vi "Multirecord Acquisition (FPGA).vi"() -> ()   [LabVIEW 2021]
doc: "Use this VI as a template for the reconfigurable oscilloscope acquisition design. The block diagram is divided into three main loops.\n\nRegister Bus: This loop initializes the registers that are needed to support the configuration of the device. The FIFO bus, on the left, allows all the other design libraries to communicate with one another. This loop is very important to support the proper behavior of the instrument design library components.\n\nAcquisition: Acquires data from the I/O channels and writes the data into the record memory using the <B>Write</B> VI of the Multirecord Acquisition instrument design library. This VI also evaluates the various acquisition triggers and decides whether to acquire each data value in record memory. The host level VI (Fetch Record.vi) can read acquired records from the DRAM. The data is stored in 2 DRAM banks, each with 768 MB of storage.\n\nFetch: The recorded data is retrieved when the <B>Fetch Single Record</B> VI is run from the host VI. The <B>Write to Fetch DMA FIFO</B> VI writes data to the acq.fetch fifo 0 to transmit record data form the FPGA to the record fetch VIs on the host. This DMA FIFO must have a predefined name based on the instance parameter. By default, it is 0 (since the associated terminal on the <B>Create Resources DRAM Write Read</B> VI is unwired), so the connected FIFO is named acq.fetch fifo 0."
uses:
  Trigger/SubVIs/Types/Trigger Type.ctl
  <instrlib>/_niInstr/Data Trigger/v1/Shared/Public/Level Configuration FXP(+-,18,1).ctl
  <instrlib>/_niInstr/Data Trigger/v1/Shared/Public/Level Configuration Trigger When.ctl
  <instrlib>/_niInstr/Data Trigger/v1/Shared/Public/Edge Configuration FXP(+-,18,1).ctl
  <instrlib>/_niInstr/Data Trigger/v1/Shared/Public/Edge Configuration Trigger Slope.ctl
  FPGA Interface Typedefinitions/Trigger Combination Type.ctl
  <vilib>/Platform/TimedLoop/XDataNode/timing_clust.ctl
  <vilib>/Platform/TimedLoop/XDataNode/nitl_modes.ctl
  <vilib>/Platform/TimedLoop/XDataNode/wakeup.ctl
  <instrlib>/_niInstr/FIFO Register Bus/v1/FPGA/niInstr FIFO Register Bus v1 FPGA.lvclass
  C:/Program Files (x86)/National Instruments/LabVIEW 2021/instr.lib/_niInstr/Instruction Framework/v1/FPGA/Interfaces/Instruction Producer/Instruction Producer.lvclass
  <instrlib>/_niInstr/Multirecord Acquisition/Common/v1/FPGA/niInstr Multirecord Acquisition Common v1 FPGA.lvclass
  C:/Program Files (x86)/National Instruments/LabVIEW 2021/instr.lib/_niInstr/Multirecord Acquisition/Interface/v1/FPGA/niInstr Multirecord Acquisition v1 FPGA.lvclass
  <vilib>/rvi/Emulation/niFpgaSctlEmulationGetInTimedLoop.vi
  <vilib>/rvi/Emulation/niFpgaEmulationReportErrorSimple.vi
  <vilib>/rvi/Emulation/niFpgaGetClockAttributes.vi
  <vilib>/rvi/Emulation/niFpgaCriticalErrorInLSC.vi
  <instrlib>/_niInstr/Multirecord Acquisition/Common/v1/FPGA/Private/Create Fetch DMA FIFO Resources U8x32.vi
  <instrlib>/_niInstr/Multirecord Acquisition/Common/v1/FPGA/Private/Create Resources DRAM U384x2 U768 Write Read.vi
  <instrlib>/_niInstr/Multirecord Acquisition/Interface/v1/FPGA/Private/Retrieve Record U16 Wrapper.vi
  <instrlib>/_niInstr/Multirecord Acquisition/Interface/v1/FPGA/Private/Write to Fetch DMA FIFO U16 Wrapper.vi
  <vilib>/rvi/eio/common/nirviEmuTemplateMethod_errors.vi
  <instrlib>/HSAI-RIO/Config/Group A/v1/FPGA/Digital Correction/Validate 8 Channel Data.vi
  <instrlib>/HSAI-RIO/Config/Group A/v1/FPGA/Digital Correction/Digital Correction (8 Ch).vi
  <instrlib>/HSAI-RIO/Config/Group A/v1/FPGA/Digital Correction/FIR Filter (8 Ch).vi
  DSP/SubVIs/Integer decimationx8ch.vi
  Data Type Conversion/SubVIs/Remove Overflow FXP(+-,18,1)x8ch.vi
  <instrlib>/_niInstr/Channel/v1/FPGA/Private/Select/Select FXP(+-,18,1,)xNspcx8ch.vi
  Trigger/Trigger FXP(+,-,18,1).vi
  Data Type Conversion/SubVIs/Data Type Conversion FXP(+-,18,1) to I16x8ch.vi
  <instrlib>/_niInstr/Channel/v1/FPGA/Private/Select and Interleave/Select And Interleave I16xNspcx8ch.vi
  <instrlib>/_niInstr/Multirecord Acquisition/Interface/v1/FPGA/Private/Write I16 Wrapper.vi
  <vilib>/Platform/TimedLoop/XDataNode/XDataNode.xnode
  <vilib>/eio/EIONode/EIONode.xnode
  <instrlib>/_niInstr/Instruction Framework/v1/FPGA/Top Level Bus/Register Configuration/Register Configuration.lvclass
  <vilib>/Platform/TimedLoop/XDataNode/XDNodeRunTimeDep.lvlib
  <instrlib>/_niInstr/Multirecord Acquisition/Interface/v1/FPGA/niInstr Multirecord Acquisition v1 FPGA.lvclass
  <vilib>/rvi/LocalResourceManager/LocalResourceManager.xnode
  <vilib>/rvi/eio/common/nirviEmuReportErrorAndStop.vi
  <vilib>/rvi/DataTransferAndStorage/Container/Common/niFpgaContainerGetUniqueNameForEmu.vi
  <vilib>/rvi/DataTransferAndStorage/Container/Common/niFpgaContainerSetEmuInfo.vi
  <instrlib>/_niInstr/Channel/v1/FPGA/niInstr Channel v1 FPGA.lvlib
  <instrlib>/_niInstr/Basic Elements/v1/FPGA/niInstr Basic Elements v1 FPGA.lvlib
  <instrlib>/HSAI-RIO/Config/Group A/v1/FPGA/Digital Correction/Digital Correction.lvclass
  <instrlib>/HSAI-RIO/Config/Group A/v1/FPGA/Config Registers/Config Registers.lvclass
  <instrlib>/_niInstr/Data Trigger/v1/Shared/niInstr Data Trigger v1 Shared.lvlib
  Emulation/SubVIs/2 Element Generate Sine Cos Data FXP(+,-,14,1).vi
  C:/Program Files (x86)/National Instruments/LabVIEW 2021/instr.lib/_niInstr/Multirecord Acquisition/Common/v1/FPGA/niInstr Multirecord Acquisition Common v1 FPGA.lvclass
  <instrlib>/_niInstr/Multirecord Acquisition/Common/v1/FPGA/Private/Create Resources BRAM U384.vi
  <instrlib>/_niInstr/Multirecord Acquisition/Common/v1/FPGA/Private/Create Resources DRAM U384.vi
  <instrlib>/_niInstr/Multirecord Acquisition/Common/v1/FPGA/Private/Create Resources BRAM U768.vi
  FPGA Interface Typedefinitions/FPGA Interface Typedefinitions.lvlib
panel:
  in  "trigger.channel A":u8
  in  "trigger.rearm delay":u16=2
  in  "start trigger":bool=TRUE
  in  "reset":bool
  in  "trigger.combination type":T1
  in  "trigger.level B":T2
  in  "trigger.edge A":T4
  in  "trigger.level A":T2
  in  "trigger.type A":T6
  out "fifo reg bus data 0":u64
  out "fifo reg bus status 0":u32
  in  "fifo reg bus ctrl 0":u32
  out "overflow":bool
  in  "dsp.decimation factor":u16
  out "overload":bool
  in  "channel.enable mask":u16=65535 format="%.0b"
  in  "channel.number of channels":u8=8
  # "Register Bus Controls"
  # "FPGA"
  # "Acquisition Loop Controls"
  # "DSP"
  # "Trigger"
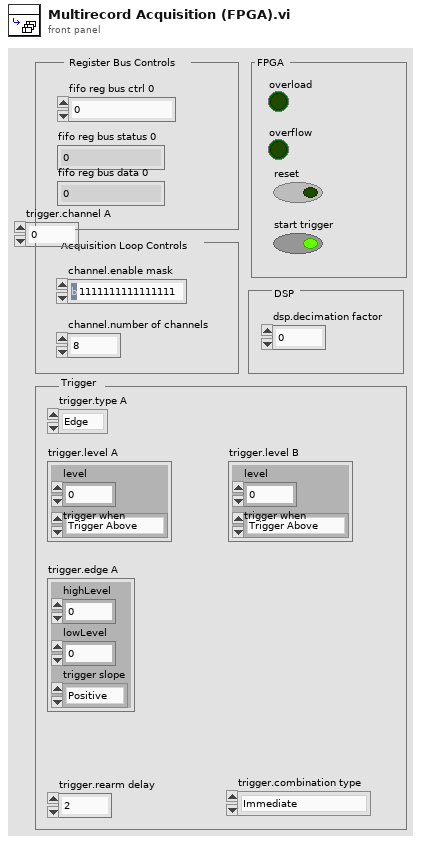
[diagram p1: front panel]
types:
  T1 = typedef "FPGA Interface Typedefinitions.lvlib/Trigger Combination Type.ctl" = enum16{"Immediate", "A", "B", "OR", "AND", "A THEN B", "B THEN A", "High Resolution"}
  T2 = typedef "niInstr Data Trigger v1 Shared.lvlib/Level Configuration FXP(+-,18,1).ctl" = cluster{"level":fxp<+/-,18,1>, "trigger when":T3}
  T3 = typedef "niInstr Data Trigger v1 Shared.lvlib/Level Configuration Trigger When.ctl" = enum8{"Trigger Above", "Trigger Below"}
  T4 = typedef "niInstr Data Trigger v1 Shared.lvlib/Edge Configuration FXP(+-,18,1).ctl" = cluster{"highLevel":fxp<+/-,18,1>, "lowLevel":fxp<+/-,18,1>, "trigger slope":T5}
  T5 = typedef "niInstr Data Trigger v1 Shared.lvlib/Edge Configuration Trigger Slope.ctl" = enum8{"Positive", "Negative"}
  T6 = typedef "Trigger Type.ctl" = enum16{"Edge", "Level", "Custom"}
  T7 = cluster{"memory 1":refnum<k21>, "memory 2":refnum<k21>}
  T8 = typedef "XDNodeRunTimeDep.lvlib/timing_clust.ctl" = cluster{"Expected End [f-1]":u64, "Actual End [f-1]":u64, "Finished Late? [f-1]":bool, "Expected End [i-1]":u64, "Actual End [i-1]":u64, "Finished Late? [i-1]":bool, "Expected Start [i]":u64, "Actual Start [i]":u64, "Expected Start [f]":u64, "Actual Start [f]":u64, "Source Name":string, "Structure Name":string, "Period":i64, "Deadline":i64, "Offset":i64, "Start":i64, "Priority":i32, "Timeout":i32, "Mode":T9, "Wakeup Reason":T10, "Error":errorcluster, "Source Type":string, "Secondary Source Type":string, "Global End Time":u64, "Global Start Time":u64, "Frame Duration":u64, "Iteration Duration":u64, "Assigned CPU":i32, "I/O Scan Engine Mode":u32}
  T9 = typedef "XDNodeRunTimeDep.lvlib/nitl_modes.ctl" = enum32{"No Change", "Process missed periods, maintain original phase", "Discard missed periods, maintain original phase", "Process missed periods, ignore original phase", "Discard missed periods, ignore original phase"}
  T10 = typedef "XDNodeRunTimeDep.lvlib/wakeup.ctl" = enum32{"Normal", "Aborted", "Asynchronous wakeup", "Timing source error", "Timed loop error", "Timeout"}
  T11 = cluster{"Channel 0":fxp<+/-,14,1>[], "Channel 1":fxp<+/-,14,1>[], "Channel 2":fxp<+/-,14,1>[], "Channel 3":fxp<+/-,14,1>[], "Channel 4":fxp<+/-,14,1>[], "Channel 5":fxp<+/-,14,1>[], "Channel 6":fxp<+/-,14,1>[], "Channel 7":fxp<+/-,14,1>[]}
  T12 = cluster{"Channel 0":fxp<+/-,18,1>[], "Channel 1":fxp<+/-,18,1>[], "Channel 2":fxp<+/-,18,1>[], "Channel 3":fxp<+/-,18,1>[], "Channel 4":fxp<+/-,18,1>[], "Channel 5":fxp<+/-,18,1>[], "Channel 6":fxp<+/-,18,1>[], "Channel 7":fxp<+/-,18,1>[]}
  T13 = cluster{"channel 0":fxp<+/-,18,1>[], "channel 1":fxp<+/-,18,1>[], "channel 2":fxp<+/-,18,1>[], "channel 3":fxp<+/-,18,1>[], "channel 4":fxp<+/-,18,1>[], "channel 5":fxp<+/-,18,1>[], "channel 6":fxp<+/-,18,1>[], "channel 7":fxp<+/-,18,1>[]}
  T14 = cluster{"channel 0":i16[], "channel 1":i16[], "channel 2":i16[], "channel 3":i16[], "channel 4":i16[], "channel 5":i16[], "channel 6":i16[], "channel 7":i16[]}
  T15 = typedef "niInstr Multirecord Acquisition v1 FPGA.lvclass/Timestamp.ctl" = cluster{"timestamp":u64, "valid":bool}
  T16 = typedef "niInstr Types v1 Shared.lvlib/Input Triggers.ctl" = cluster{"start":bool, "advance":bool, "reference":bool, "start trigger index":u16, "advance trigger index":u16, "reference trigger index":u16, "reference trigger correction cycle count":u32}
  T17 = typedef "niInstr Types v1 Shared.lvlib/Sample Format.ctl" = cluster{"bits per channel":u16, "samples per clock":u16, "channels":u8}
  T18 = typedef "niInstr Multirecord Acquisition v1 FPGA.lvclass/Events.ctl" = cluster{"ready for start":bool, "ready for advance":bool, "ready for reference":bool, "end of record":bool, "done":bool, "start trigger":bool, "advance trigger":bool, "reference trigger":bool, "start trigger index":u16, "advance trigger index":u16, "reference trigger index":u16}
  T19 = typedef "niInstr Multirecord Acquisition v1 FPGA.lvclass/Retrieve Data Info.ctl" = cluster{"read request size (bits)":u64, "valid data offset (bits)":u16, "valid data size (bits)":u16, "first sample of request":bool, "last sample of request":bool, "Token":T20}
  T20 = typedef "niInstr Types v1 Shared.lvlib/Token.ctl" = cluster{"identifier":u8, "value":u32}
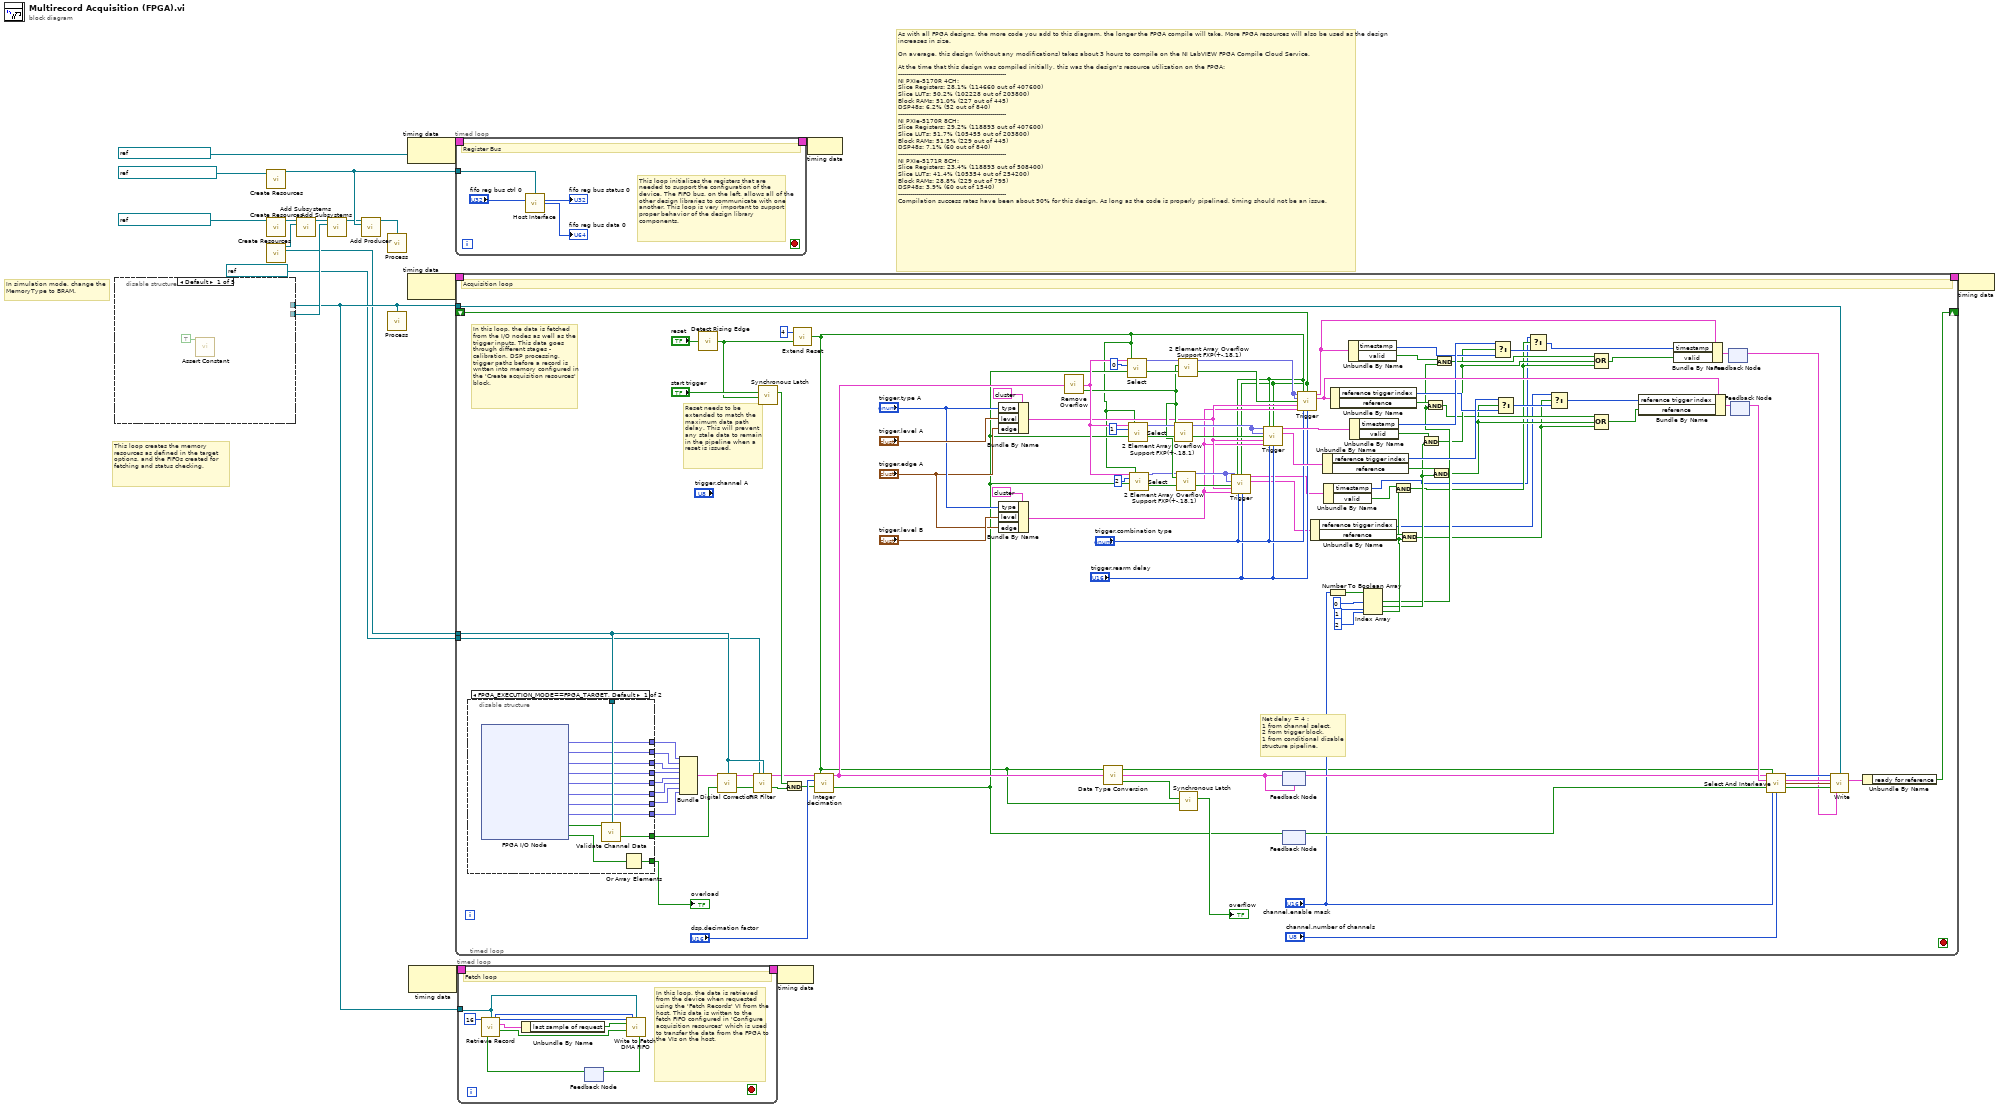
[diagram p0: block diagram]
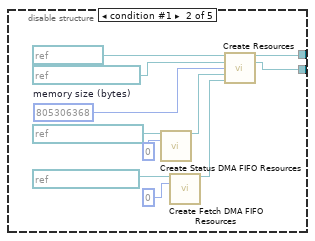
[diagram p2: hidden frame]
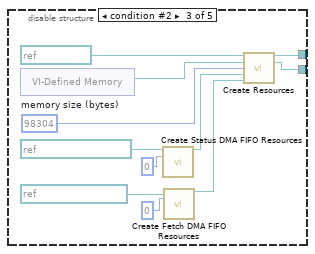
[diagram p3: hidden frame]
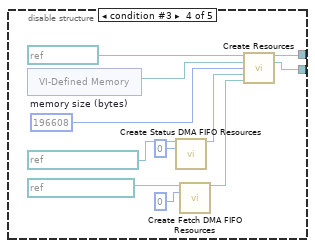
[diagram p4: hidden frame]
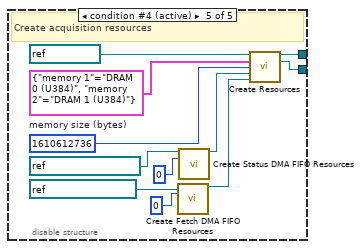
[diagram p5: hidden frame]
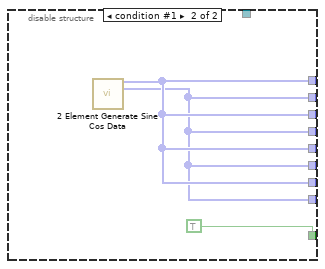
[diagram p6: hidden frame]
diagram:
  # "In simulation mode, change the MemoryType to BRAM."
  # "This loop creates the memory resources as defined in the target options, and the FIFOs created for fetching and status checking."
  # "As with all FPGA designs, the more code you add to this diagram, the longer the FPGA compile will take. More FPGA resources will also be used as the design increases in size.\n\nOn average, this design (without any modifications) takes about 3 hours to compile on the NI LabVIEW FPGA Compile Cloud Service. \n\nAt the time that this design was compiled initially, this was the design's resource utilization on the FPGA:\n------------------------------------------------------\nNI PXIe-5170R 4CH:\nSlice Registers: 28.1% (114660 out of 407600)\nSlice LUTs: 50.2% (102228 out of 203800)\nBlock RAMs: 51.0% (227 out of 445)\nDSP48s: 6.2% (52 out of 840)\n------------------------------------------------------\nNI PXIe-5170R 8CH:\nSlice Registers: 29.2% (118893 out of 407600)\nSlice LUTs: 51.7% (105455 out of 203800)\nBlock RAMs: 51.5% (229 out of 445)\nDSP48s: 7.1% (60 out of 840)\n------------------------------------------------------\nNI PXIe-5171R 8CH:\nSlice Registers: 23.4% (118893 out of 508400)\nSlice LUTs: 41.4% (105354 out of 254200)\nBlock RAMs: 28.8% (229 out of 795)\nDSP48s: 3.9% (60 out of 1540)\n------------------------------------------------------\nCompilation success rates have been about 90% for this design. As long as the code is properly pipelined, timing should not be an issue."
  n1 = disable-structure shown="Default" {
    disable-tunnel: [_ w29 w40 w51 w62] -> w4
    disable-tunnel: [_ w26 w36 w47 w59] -> w7
    frame condition #0 {
      n2 = call <instrlib>:"Assert Constant.vi"("constant terminal"=TRUE) -> ()  [unwired: 15 in]
    }
    frame condition #1 {
      w30 = u64 805306368  # memory size (bytes)
      n3 = call <instrlib>:"Create Status DMA FIFO Resources.vi"("status dma fifo in"=refnum<k21> "acq.status fifo 0" ("status dma fifo"), "fifo instance"=u8 0) -> ("status dma fifo out"=w21:refnum<class "niInstr Status FIFO v1 FPGA.lvclass">)  [unwired: 13 in]
      n4 = call-poly <instrlib>:"Create Fetch DMA FIFO Resources.vi"("fetch dma fifo in"=refnum<k21> "acq.fetch fifo 0", "fifo instance"=u8 0) -> ("fetch dma fifo out"=w27:refnum<class "niInstr Fetch FIFO v1 FPGA.lvclass">)  [unwired: 13 in]
      n5 = call-poly <instrlib>:"Create Resources.vi"("memory clock"=refnum<k21> "160MHz" ("process clock"), "memory"=refnum<k21> "DRAM 0 (U384)" ("dram"), "memory size (bytes)"=w30, "status dma fifo resources"=w21, "fetch dma fifo resources"=w27) -> ("acquisition resources"=w29:refnum<class "niInstr Multirecord Acquisition Common v1 FPGA.lvclass">, "acquisition subsystem"=w26:refnum<class "Address Space Collection.lvclass">)  [unwired: 9 in]
    }
    frame condition #2 {
      w41 = u64 98304  # memory size (bytes)
      n6 = xnode "VI-Defined Memory"() -> ("Memory Out"=w42:refnum<k21>)
      n7 = call <instrlib>:"Create Status DMA FIFO Resources.vi"("status dma fifo in"=refnum<k21> "acq.status fifo 0" ("status dma fifo"), "fifo instance"=u8 0) -> ("status dma fifo out"=w33:refnum<class "niInstr Status FIFO v1 FPGA.lvclass">)  [unwired: 13 in]
      n8 = call-poly <instrlib>:"Create Fetch DMA FIFO Resources.vi"("fetch dma fifo in"=refnum<k21> "acq.fetch fifo 0", "fifo instance"=u8 0) -> ("fetch dma fifo out"=w37:refnum<class "niInstr Fetch FIFO v1 FPGA.lvclass">)  [unwired: 13 in]
      n9 = call-poly <instrlib>:"Create Resources.vi"("memory clock"=refnum<k21> "160MHz" ("process clock"), "memory"=w42, "memory size (bytes)"=w41, "status dma fifo resources"=w33, "fetch dma fifo resources"=w37) -> ("acquisition resources"=w40:refnum<class "niInstr Multirecord Acquisition Common v1 FPGA.lvclass">, "acquisition subsystem"=w36:refnum<class "Address Space Collection.lvclass">)  [unwired: 9 in]
    }
    frame condition #3 {
      w52 = u64 196608  # memory size (bytes)
      n10 = xnode "VI-Defined Memory"() -> ("Memory Out"=w53:refnum<k21>)
      n11 = call <instrlib>:"Create Status DMA FIFO Resources.vi"("status dma fifo in"=refnum<k21> "acq.status fifo 0" ("status dma fifo"), "fifo instance"=u8 0) -> ("status dma fifo out"=w45:refnum<class "niInstr Status FIFO v1 FPGA.lvclass">)  [unwired: 13 in]
      n12 = call-poly <instrlib>:"Create Fetch DMA FIFO Resources.vi"("fetch dma fifo in"=refnum<k21> "acq.fetch fifo 0", "fifo instance"=u8 0) -> ("fetch dma fifo out"=w48:refnum<class "niInstr Fetch FIFO v1 FPGA.lvclass">)  [unwired: 13 in]
      n13 = call-poly <instrlib>:"Create Resources.vi"("memory clock"=refnum<k21> "160MHz" ("process clock"), "memory"=w53, "memory size (bytes)"=w52, "status dma fifo resources"=w45, "fetch dma fifo resources"=w48) -> ("acquisition resources"=w51:refnum<class "niInstr Multirecord Acquisition Common v1 FPGA.lvclass">, "acquisition subsystem"=w47:refnum<class "Address Space Collection.lvclass">)  [unwired: 9 in]
    }
    frame condition #4 (active) {
      w64 = u64 1610612736  # memory size (bytes)
      # "Create acquisition resources"
      n14 = call-poly <instrlib>:"Create Fetch DMA FIFO Resources.vi"("fetch dma fifo in"=refnum<k21> "acq.fetch fifo 0", "fifo instance"=u8 0) -> ("fetch dma fifo out"=w61:refnum<class "niInstr Fetch FIFO v1 FPGA.lvclass">)  [unwired: 13 in]
      n15 = call <instrlib>:"Create Status DMA FIFO Resources.vi"("status dma fifo in"=refnum<k21> "acq.status fifo 0" ("status dma fifo"), "fifo instance"=u8 0) -> ("status dma fifo out"=w56:refnum<class "niInstr Status FIFO v1 FPGA.lvclass">)  [unwired: 13 in]
      n16 = call-poly <instrlib>:"Create Resources.vi"("memory clock"=refnum<k21> "160MHz" ("process clock"), "memory"=T7 {"memory 1"="DRAM 0 (U384)", "memory 2"="DRAM 1 (U384)"}, "memory size (bytes)"=w64, "status dma fifo resources"=w56, "fetch dma fifo resources"=w61) -> ("acquisition resources"=w62:refnum<class "niInstr Multirecord Acquisition Common v1 FPGA.lvclass">, "acquisition subsystem"=w59:refnum<class "Address Space Collection.lvclass">)  [unwired: 9 in]
    }
  }
  n17 = call <instrlib>:"Create Resources.vi"("instruction fifo"=refnum<k21> "reg.host instruction fifo 0" ("FIFO")) -> ("fifo register bus"=w6:refnum<class "niInstr FIFO Register Bus v1 FPGA.lvclass">)  [unwired: 14 in]
  n18 = call <instrlib>:"Create Resources.vi"("register clock"=refnum<k21> "40 MHz Onboard Clock" ("Source Name")) -> ("register configuration"=w10:refnum<class "Register Configuration.lvclass">)  [unwired: 14 in]
  n19 = call <instrlib>:"Create Resources.vi"() -> ("config subsystems"=w8:refnum<class "Address Space Collection.lvclass">, "digital correction resources"=w1:refnum<class "Digital Correction.lvclass">)  [unwired: 14 in]
  n20 = call-dynamic "Add Subsystems.vi"("register configuration in"=w10, "subsystems"=w8) -> ("register configuration out"=w9:refnum<class "Register Configuration.lvclass">)  [unwired: 13 in]
  n21 = call-dynamic "Add Subsystems.vi"("register configuration in"=w9, "subsystems"=w7) -> ("register configuration out"=w3:refnum<class "Register Configuration.lvclass">)  [unwired: 13 in]
  n22 = call-dynamic "Add Producer.vi"("register configuration in"=w3, "instruction producer"=w6) -> ("register configuration out"=w5:refnum<class "Register Configuration.lvclass">)  [unwired: 13 in]
  n23 = call-dynamic "Process.vi"("register configuration"=w5) -> ()  [unwired: 15 in]
  n24 = call-dynamic "Process.vi"("acquisition resources"=w4) -> ()  [unwired: 15 in]
  n25 = node-c288(refnum<k21> "40 MHz Onboard Clock" ("Source Name")) -> (w19:T8)
  n26 = node-c288() -> (w17:T8)  [unwired: 1 in]
  n27 = node-c288() -> (w15:T8)  [unwired: 1 in]
  n28 = timed-loop {
    timing: w19 -> [_]
    timing-out: [_] -> w18
    tunnel: w6 -> [w68]
    stop <- _ stop-if-true
    # "This loop initializes the registers that are needed to support the configuration of the device. The FIFO bus, on the left, allows all of the other design libraries to communicate with one another. This loop is very important to support proper behavior of the design library components."
    # "Register Bus"
    n29 = call <instrlib>:"Host Interface.vi"("fifo register bus"=w68, "fifo reg bus ctrl 0"="fifo reg bus ctrl 0") -> ("fifo reg bus status 0"=→"fifo reg bus status 0":u32, "fifo reg bus data 0"=→"fifo reg bus data 0":u64)  [unwired: 12 in]
  }
  n30 = timed-loop {
    timing: w17 -> [_]
    timing-out: [_] -> w16
    tunnel: w4 -> [w176]
    tunnel: w1 -> [w155]
    shift-right: [w168] -> _
    shift-left: _ -> [w92]
    tunnel: refnum<k21> "Data Clock x2" -> [w152]
    stop <- _ stop-if-true
    # "Net delay = 4 :\n1 from channel select.\n2 from trigger block.\n1 from conditional disable structure pipeline."
    # "Reset needs to be extended to match the maximum data path delay. This will prevent any stale data to remain in the pipeline when a reset is issued."
    # "In this loop, the data is fetched from the I/O nodes as well as the trigger inputs. This data goes through different stages - calibration, DSP processing, trigger paths before a record is written into memory configured in the 'Create acquisition resources' block."
    # "Acquisition loop"
    n31 = disable-structure shown="FPGA_EXECUTION_MODE==FPGA_TARGET, Default" {
      disable-tunnel: [w188 w193] -> w151
      disable-tunnel: [w187 w192] -> w150
      disable-tunnel: [w186 w193] -> w149
      disable-tunnel: [w185 w192] -> w148
      disable-tunnel: [w184 w193] -> w147
      disable-tunnel: [w183 w192] -> w146
      disable-tunnel: [w182 w193] -> w144
      disable-tunnel: [w181 w192] -> w145
      disable-tunnel: [w178 TRUE ("ADC Data Valid")] -> w142
      disable-tunnel: w155 -> [w189 _]
      disable-tunnel: [w179 _] -> w175
      frame condition #0 (active) {
        # "I/O Nodes"
        n32 = xnode "FPGA I/O Node"() -> ("Channel 0"=w188:fxp<+/-,14,1>[], "Channel 1"=w187:fxp<+/-,14,1>[], "Channel 2"=w186:fxp<+/-,14,1>[], "Channel 3"=w185:fxp<+/-,14,1>[], "Channel 4"=w184:fxp<+/-,14,1>[], "Channel 5"=w183:fxp<+/-,14,1>[], "Channel 6"=w182:fxp<+/-,14,1>[], "Channel 7"=w181:fxp<+/-,14,1>[], "Channel Data Valid"=w190:bool[], "Channel Overload"=w180:bool[])  [unwired: 10 in, 10 out]
        n33 = call-poly <instrlib>:"Validate Channel Data.vi"("channel data valid"=w190, "digital correction resources"=w189) -> ("expected data valid"=w178:bool)  [unwired: 13 in]
        n34 = Or Array Elements(Boolean array=w180) -> (logical OR=w179:bool)
      }
      frame condition #1 {
        n35 = call-poly "2 Element Generate Sine Cos Data.vi"() -> ("sine data"=w193:fxp<+/-,14,1>[], "cosine data"=w192:fxp<+/-,14,1>[])  [unwired: 14 in]
      }
    }
    "overload" <- w175
    n36 = Bundle("Channel 0"=w151, "Channel 1"=w150, "Channel 2"=w149, "Channel 3"=w148, "Channel 4"=w147, "Channel 5"=w146, "Channel 6"=w144, "Channel 7"=w145) -> (w143:T11)  [unwired: 1 in]
    n37 = call <instrlib>:"Detect Rising Edge.vi"("signal"="reset") -> ("edge detected"=w154:bool)  [unwired: 14 in]
    n38 = call-poly <instrlib>:"Digital Correction.vi"("channel data in"=w143, "digital correction resources"=w155, "input valid"=w142) -> ("corrected channel data out"=w135:T12, "output valid"=w134:bool)  [unwired: 11 in]
    n39 = call-poly <instrlib>:"FIR Filter.vi"("data in"=w135, "data clock x2"=w152, "digital correction resources"=w155, "input valid"=w134) -> ("data out"=w132:T12, "output valid"=w133:bool)  [unwired: 9 in, 1 out]
    n40 = call <instrlib>:"Synchronous Latch.vi"("clear"=w154, "set"="start trigger") -> ("out"=w160:bool)  [unwired: 9 in]
    n41 = And(x=w160, y=w133) -> (x .and. y?=w136:bool)
    n42 = call "Extend Reset.vi"("reset in"=w154, "number of cycles"=u8 4) -> ("reset out"=w93:bool)
    n43 = call-poly "Integer decimation.vi"("data in"=w132, "reset"=w93, "decimation factor"="dsp.decimation factor", "input valid"=w136) -> ("data out"=w139:T13, "output valid"=w102:bool)  [unwired: 9 in, 1 out]
    n44 = Bundle By Name(cluster=cluster{"type":T6, "level":T2, "edge":T4} {"type"=enum."Edge", "level"={"level"=0.0, "trigger when"=enum."Trigger Above"}, "edge"={"highLevel"=0.0, "lowLevel"=0.0, "trigger slope"=enum."Positive"}} ("trigger.A"), "type"="trigger.type A", "level"="trigger.level A", "edge"="trigger.edge A") -> (w97:cluster{"type":T6, "level":T2, "edge":T4})
    n45 = Bundle By Name(cluster=cluster{"type":T6, "level":T2, "edge":T4} {"type"=enum."Edge", "level"={"level"=0.0, "trigger when"=enum."Trigger Above"}, "edge"={"highLevel"=0.0, "lowLevel"=0.0, "trigger slope"=enum."Positive"}} ("trigger.A"), "type"="trigger.type A", "level"="trigger.level B", "edge"="trigger.edge A") -> (w96:cluster{"type":T6, "level":T2, "edge":T4})
    n46 = call-poly "Remove Overflow.vi"("data in"=w139) -> ("overflow"=w101:bool, "data out"=w104:T13)  [unwired: 3 in]
    n47 = call-poly "Data Type Conversion.vi"("data in"=w139) -> ("overflow"=w141:bool, "data out"=w138:T14)  [unwired: 3 in]
    n48 = call-poly <instrlib>:"Select.vi"("data in"=w104, "reset"=w93, "channel index"=u8 0 ("trigger.channel A"), "input valid"=w102) -> ("channel out"=w162:fxp<+/-,18,1>[], "output valid"=w131:bool)  [unwired: 10 in]
    n49 = call-poly <instrlib>:"Select.vi"("data in"=w104, "reset"=w93, "channel index"=u8 1, "input valid"=w102) -> ("channel out"=w126:fxp<+/-,18,1>[], "output valid"=w124:bool)  [unwired: 10 in]
    n50 = call-poly <instrlib>:"Select.vi"("data in"=w104, "reset"=w93, "channel index"=u8 2, "input valid"=w102) -> ("channel out"=w100:fxp<+/-,18,1>[], "output valid"=w98:bool)  [unwired: 10 in]
    n51 = call "2 Element Array Overflow Support FXP(+-,18,1).vi"("data in"=w126, "overflow"=w101) -> ("data out"=w125:fxp<+/-,18,1>[])  [unwired: 13 in]
    n52 = call "2 Element Array Overflow Support FXP(+-,18,1).vi"("data in"=w100, "overflow"=w101) -> ("data out"=w99:fxp<+/-,18,1>[])  [unwired: 13 in]
    n53 = call "2 Element Array Overflow Support FXP(+-,18,1).vi"("data in"=w162, "overflow"=w101) -> ("data out"=w130:fxp<+/-,18,1>[])  [unwired: 13 in]
    n54 = call <instrlib>:"Synchronous Latch.vi"("clear"=w93, "set"=w141) -> ("out"=→"overflow":bool)  [unwired: 9 in]
    n55 = call-poly "Trigger.vi"("data A"=w99, "reset"=w93, "trigger.ready for reference"=w92, "data B"=w99, "input valid"=w98, "trigger.A"=w97, "trigger.B"=w96, "trigger.combination type"="trigger.combination type", "rearm delay"="trigger.rearm delay") -> ("timestamps"=w91:T15, "trigger.out"=w90:T16)  [unwired: 4 in, 1 out]
    n56 = call-poly "Trigger.vi"("data A"=w125, "reset"=w93, "trigger.ready for reference"=w92, "data B"=w125, "input valid"=w124, "trigger.A"=w97, "trigger.B"=w96, "trigger.combination type"="trigger.combination type", "rearm delay"="trigger.rearm delay") -> ("timestamps"=w119:T15, "trigger.out"=w118:T16)  [unwired: 4 in, 1 out]
    n57 = feedback #1(w138) -> (w140:T14)
    n58 = feedback-in #1(w138) -> ()
    n59 = feedback #2() -> (w137:bool)  [unwired: 1 in]
    n60 = feedback-in #2(w102) -> ()
    n61 = call-poly "Trigger.vi"("data A"=w130, "reset"=w93, "trigger.ready for reference"=w92, "data B"=w130, "input valid"=w131, "trigger.A"=w97, "trigger.B"=w96, "trigger.combination type"="trigger.combination type", "rearm delay"="trigger.rearm delay") -> ("timestamps"=w123:T15, "trigger.out"=w121:T16)  [unwired: 4 in, 1 out]
    n62 = Unbundle By Name(w90) -> ("reference trigger index"=w71:u16, "reference"=w89:bool)
    n63 = Unbundle By Name(w118) -> ("reference trigger index"=w115:u16, "reference"=w106:bool)
    n64 = Unbundle By Name(w91) -> ("timestamp"=w73:u64, "valid"=w85:bool)
    n65 = Number To Boolean Array(number="channel.enable mask") -> (Boolean array=w112:bool[])
    n66 = Unbundle By Name(w121) -> ("reference trigger index"=w114:u16, "reference"=w107:bool)
    n67 = Unbundle By Name(w123) -> ("timestamp"=w116:u64, "valid"=w109:bool)
    n68 = Unbundle By Name(w119) -> ("timestamp"=w117:u64, "valid"=w108:bool)
    n69 = Index Array(array=w112, index #1=0 ("index"), index #2=1 ("index"), index #3=2 ("index")) -> (element #1=w86:bool, element #2=w87:bool, element #3=w88:bool)
    n70 = And(x=w85, y=w88) -> (x .and. y?=w74:bool)
    n71 = And(x=w89, y=w88) -> (x .and. y?=w72:bool)
    n72 = And(x=w108, y=w87) -> (x .and. y?=w83:bool)
    n73 = And(x=w107, y=w86) -> (x .and. y?=w81:bool)
    n74 = And(x=w106, y=w87) -> (x .and. y?=w80:bool)
    n75 = And(x=w109, y=w86) -> (x .and. y?=w84:bool)
    n76 = Select(t=w117, s=w83, f=w116) -> (s? t:f=w78:u64)
    n77 = Select(t=w115, s=w80, f=w114) -> (s? t:f=w76:u16)
    n78 = Select(t=w73, s=w74, f=w78) -> (s? t:f=w77:u64)
    n79 = Select(t=w71, s=w72, f=w76) -> (s? t:f=w75:u16)
    n80 = Compound Arithmetic op=OR(w84, w83, w74) -> (w82:bool)
    n81 = Compound Arithmetic op=OR(w81, w80, w72) -> (w79:bool)
    n82 = Bundle By Name(cluster=w121, "reference trigger index"=w75, "reference"=w79) -> (w120:T16)
    n83 = Bundle By Name(cluster=w123, "timestamp"=w77, "valid"=w82) -> (w122:T15)
    n84 = feedback #3() -> (w158:T15)  [unwired: 1 in]
    n85 = feedback-in #3(w122) -> ()
    n86 = feedback #4() -> (w159:T16)  [unwired: 1 in]
    n87 = feedback-in #4(w120) -> ()
    n88 = call-poly <instrlib>:"Select And Interleave.vi"("data in"=w140, "reset"=w93, "triggers in"=w159, "input valid"=w137, "channel enable mask"="channel.enable mask", "number of channels to interleave"="channel.number of channels") -> ("interleaved data out"=w174:i16[], "triggers out"=w173:T16, "sample format out"=w172:T17, "output valid"=w171:bool)  [unwired: 5 in, 1 out]
    n89 = call-poly <instrlib>:"Write.vi"("data"=w174, "acquisition resources"=w176, "triggers"=w173, "sample format"=w172, "data valid"=w171, "timestamp"=w158) -> ("events"=w169:T18)  [unwired: 6 in, 3 out]
    n90 = Unbundle By Name(w169) -> ("ready for reference"=w168:bool)
  }
  n91 = timed-loop {
    timing: w15 -> [_]
    timing-out: [_] -> w14
    tunnel: w4 -> [w204]
    stop <- _ stop-if-true
    # "In this loop, the data is retrieved from the device when requested using the 'Fetch Records' VI from the host. This data is written to the fetch FIFO configured in 'Configure acquisition resources' which is used to transfer the data from the FPGA to the VIs on the host."
    # "Fetch loop"
    n92 = feedback #5() -> (w202:bool)  [unwired: 1 in]
    n93 = call-poly <instrlib>:"Retrieve Record.vi"("output array size"=u16 16, "acquisition resources"=w204, "ready for output"=w202) -> ("channels"=w197:u8, "data"=w200:u16[], "retrieve data info"=w199:T19, "output valid"=w201:bool)  [unwired: 9 in]
    n94 = Unbundle By Name(w199) -> ("last sample of request"=w198:bool)
    n95 = call-poly <instrlib>:"Write to Fetch DMA FIFO.vi"("data"=w200, "channels"=w197, "acquisition resources"=w204, "last sample of request"=w198, "input valid"=w201) -> ("ready for input"=w203:bool)  [unwired: 10 in]
    n96 = feedback-in #5(w203) -> ()
  }
  n97 = node-c288(w14) -> ()
  n98 = node-c288(w18) -> ()
  n99 = node-c288(w16) -> ()
